vi "Burn-In Testing_v2.vi"() -> ()   [LabVIEW 2012]
uses:
  Controls/Command_Enum.ctl
  TestData/Command.ctl
  Controls/Exit.vi
  Classes/EpiWrapper.lvclass
  Controls/USB4000_Data.ctl
  Controls/Instr_Param.ctl
  Controls/PathTypes.ctl
  Controls/PathTraveler.ctl
  Controls/AppPaths.ctl
  Controls/PadArea.ctl
  Controls/Pad.ctl
  Controls/SelectedPads.ctl
  Controls/PadLookupItem.ctl
  Controls/PadLookup.ctl
  Controls/Measurement.ctl
  Controls/TestData.ctl
  Controls/MeasureControl.ctl
  Controls/MapEventType.ctl
  PadLookupVar.vi
  Controls/PadAreaItemStrings.ctl
  PadAreaStringsVar.vi
  Controls/UserInput.ctl
  Controls/MapPOS.ctl
  Controls/WaferTable.ctl
  Controls/Config.ctl
  Instruments/TypeDefs/SMUParam.ctl
  Controls/WaferSize.ctl
  Controls/CurrentPad.ctl
  Controls/MeasurementType.ctl
panel:
  in  "CurrentPad":T1
  in  "MeasureControl":T3 {"TestData"."50mA Data"."Reverse" format="%#_3g"; "TestData"."50mA Data"."Current,mA" format="%_6g"; "TestData"."50mA Data"."Knee Current" format="%#_3g"; "TestData"."50mA Data"."WL" format="%_6g"; "TestData"."50mA Data"."Voltage" format="%_6g"; "TestData"."50mA Data"."Power" format="%_5g"; "TestData"."20mA Data"."Reverse" format="%#_3g"; "TestData"."20mA Data"."Current,mA" format="%_6g"; "TestData"."20mA Data"."Knee Current" format="%#_3g"; "TestData"."20mA Data"."WL" format="%_6g"; "TestData"."20mA Data"."Voltage" format="%_6g"; "TestData"."20mA Data"."Power" format="%_5g"}
  in  "Tab Control":enum32{"Data 20mA", "Data 50mA"}(tab)
  in  "Wafer Data,20mA":T6
  in  "Wafer Data,50mA":T6
  in  "PadLookup":T7
  out "SelectedPads":T9
  out "2D Picture":picture
  out "SpectrumSat":bool
  in  "AppPaths":T11={"DataDir"={"Enum"=enum."DataDir", "FileName"="", "Exists?"=FALSE, "Path"=path ""}, "OmniDriver"={"Enum"=enum."OmniDriver", "FileName"="OmniDriver32.dll", "Exists?"=FALSE, "Path"=path ""}, "OmniDriverCommon"={"Enum"=enum."OmniDriver_Common", "FileName"="common32.dll", "Exists?"=FALSE, "Path"=path ""}, "Configuration"={"Enum"=enum."Configuration", "FileName"="TestConfiguration.cfg", "Exists?"=FALSE, "Path"=path ""}, "WaferImage"={"Enum"=enum."WaferImage", "FileName"="EPI_Wafer_Labels.jpg", "Exists?"=FALSE, "Path"=path ""}}
  in  "Configuration":T14={"IntTime"=100, "Samples"=3, "PowerMin"=300.0, "KneeMin"=-20.0, "KneeMax"=20.0, "Background Wl"=275.0, "Settle Delay,ms"=275, "StationId"=0.0} {"Background Wl" min=220.0 max=320.0; "IntTime" min=1 max=100000; "Samples" min=1 max=10; "PowerMin" min=0.0 max=10000.0; "KneeMin" min=-40.0 max=0.0; "KneeMax" min=0.0 max=40.0}
  out "Output For Excel":string
  in  "Integration Time(ms)\nMin=10ms":i32=10 min=10 max=100000
  out "Status":bool
  in  "MapPOS":T15
  in  "INSTR_PARAM":T16={"Keithley_Param"={"Start Current,mA"=0.0, "Stop Current,mA"=0.0, "Voltage Compliance,V"=0.0, "GPIB"="", "VISA resource name"="GPIB0::24::INSTR"}, "USB4000_Param"={"Integration Time"=0, "Wl min,nm"=0.0, "Wl max,nm"=0.0, "USB4000"={"Wrapper Out"=0, "Number of Spectrometers"=0, "Wavelength"=[], "EL Spectrum"=[], "Int Time (usec)"=0, FALSE, "Background"=[]}}, "Ophir_Param"={"VISA resource name"="", "Calibration Wl"=0.0}}
  in  "Stop":bool
  in  "Input":T19={"Wafer ID"="", "Test Type"=enum."Initial", "New"=FALSE, "Save"=FALSE, "Load"=FALSE, "Cancel"=FALSE, "Wafer Size"="2"}
  # "Quick Test"
  # "Measure Control"
  # "Measurement Settings"
  # "Test Criteria"
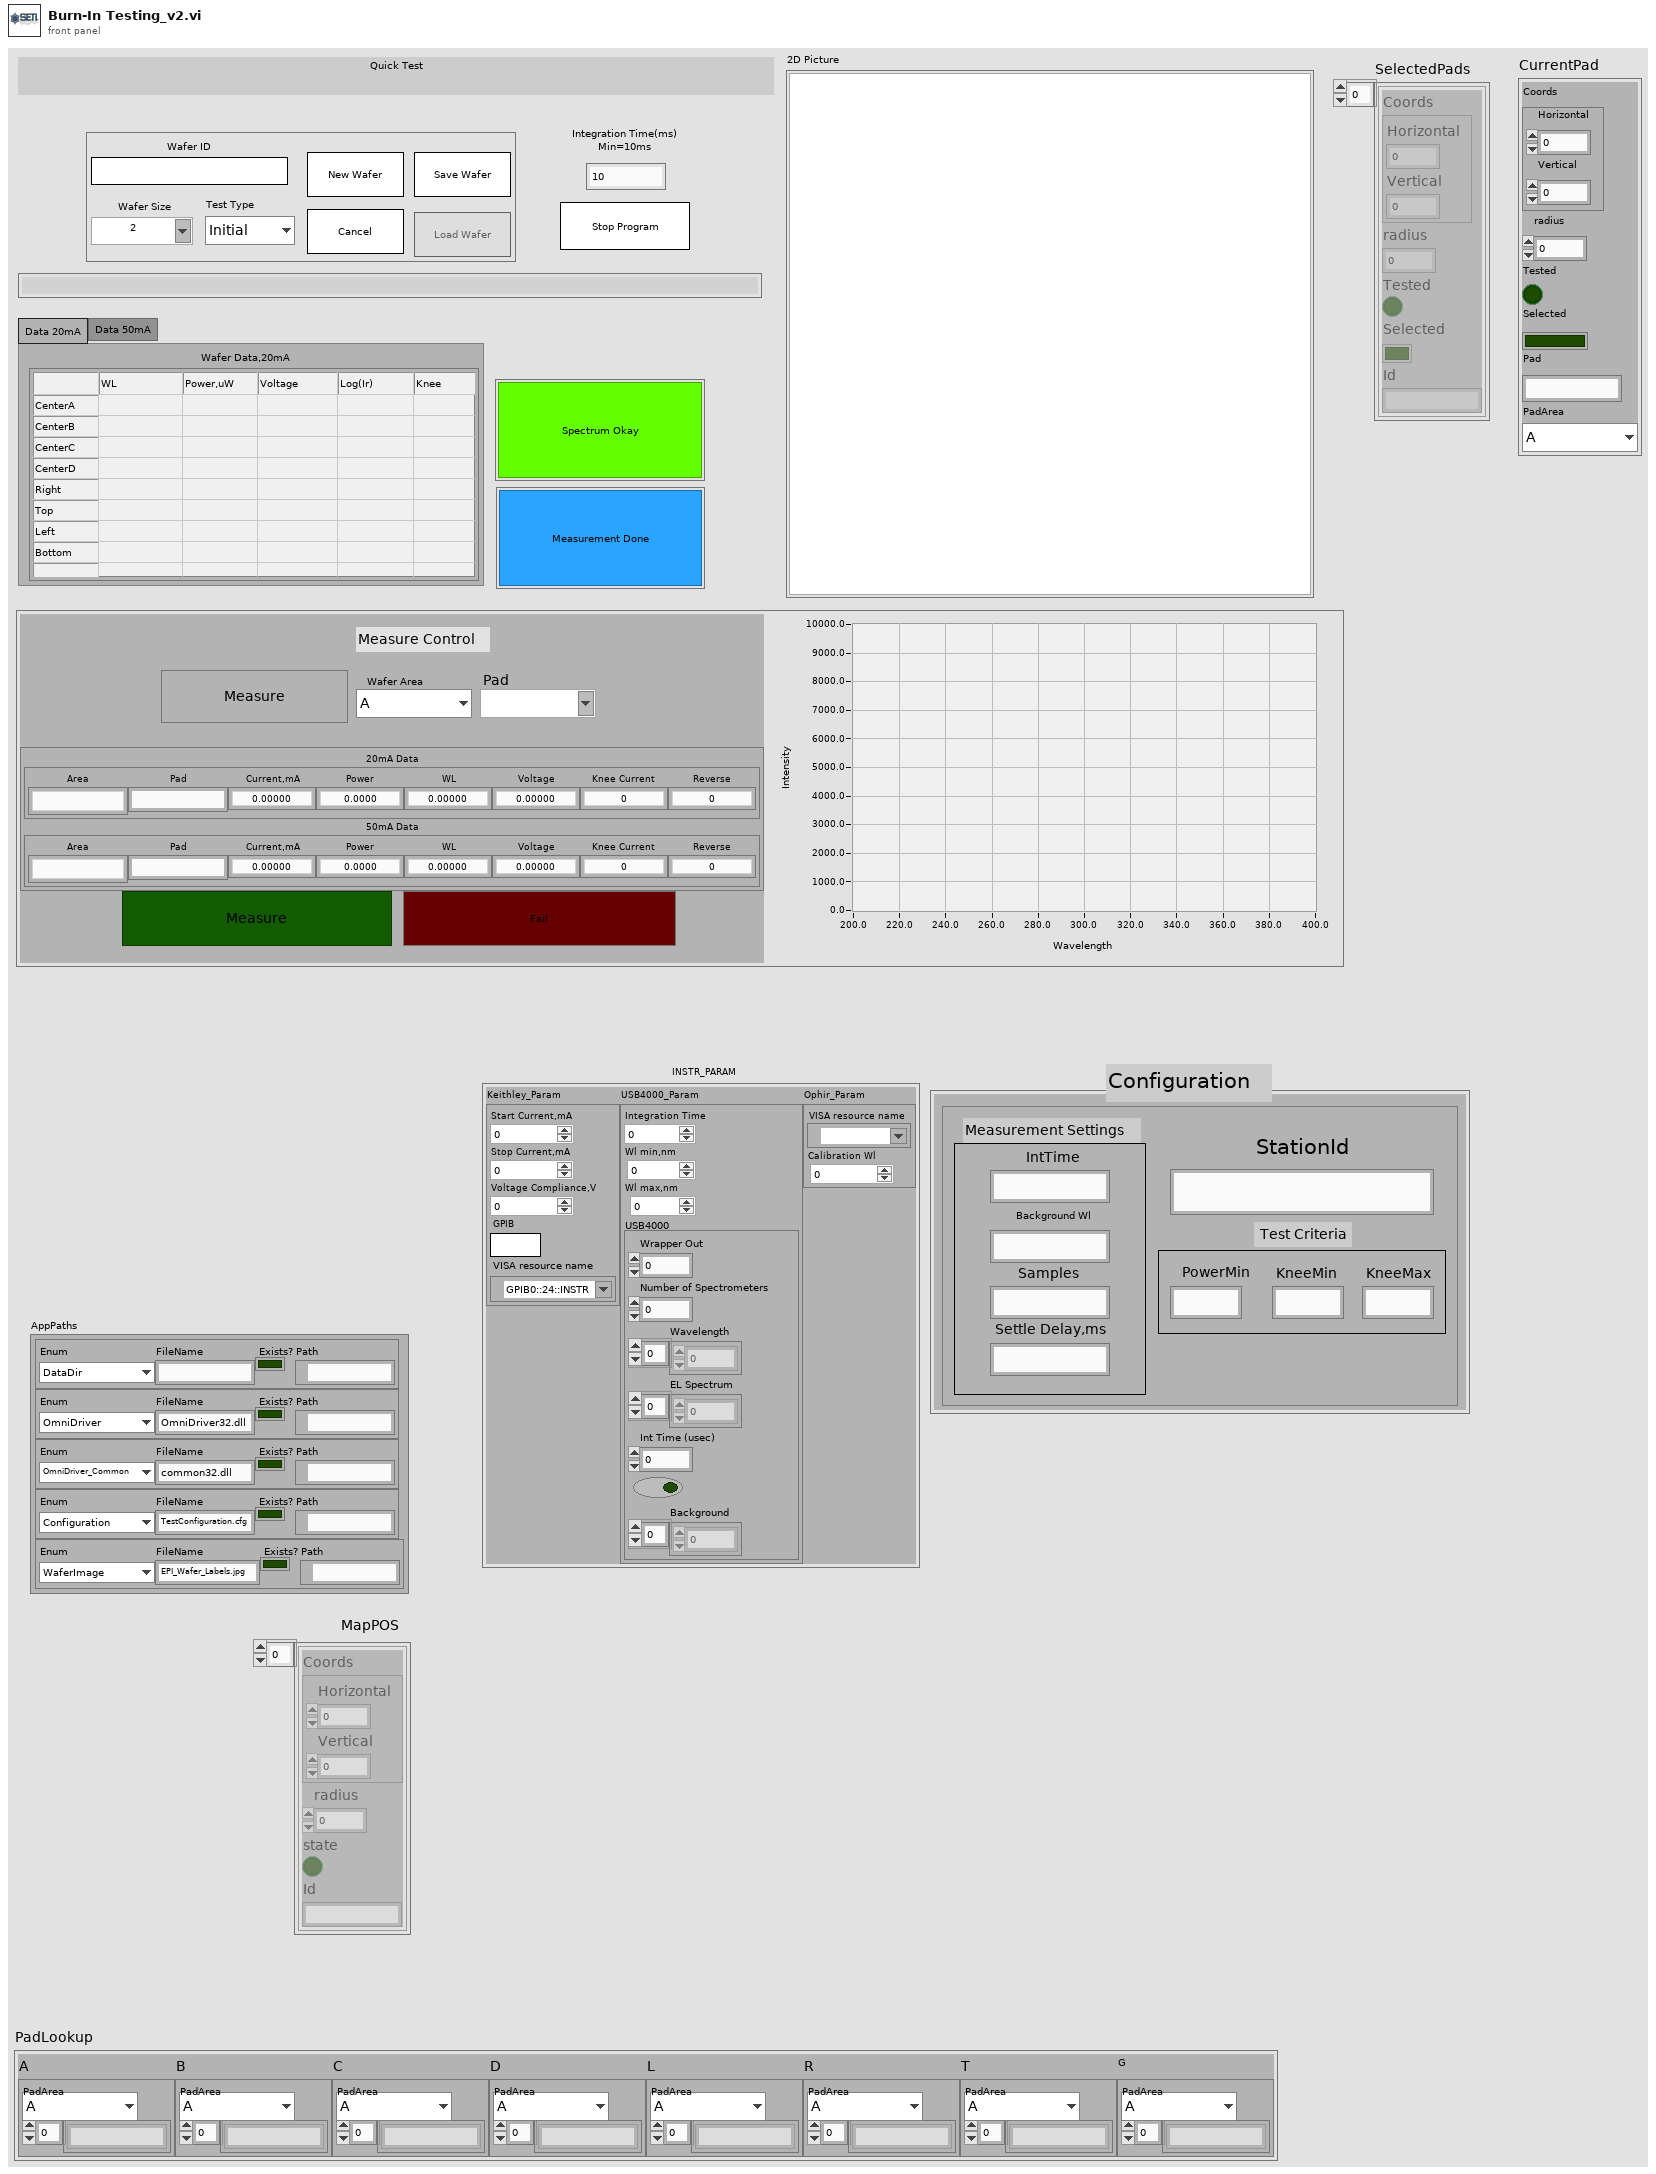
[diagram p1: front panel]
types:
  T1 = typedef "CurrentPad.ctl" = cluster{"Coords":cluster{"Horizontal":sgl, "Vertical":sgl}, "radius":i32, "Tested":bool, "Selected":bool, "Pad":string, "PadArea":T2}
  T2 = typedef "PadArea.ctl" = enum16{"A", "B", "C", "D", "L", "R", "T", "G"}
  T3 = typedef "MeasureControl.ctl" = cluster{"Graph":cluster{"Y":dbl[], "Y":dbl[]}[], "Pass":bool, "Fail":bool, "Measure":bool, "Wafer Area":T2, "TestData":T4, "Pad":string}
  T4 = typedef "TestData.ctl" = cluster{"20mA Data":T5, "50mA Data ":T5}
  T5 = typedef "Measurement.ctl" = cluster{"Area":string, "Pad":string, "Current,mA":dbl, "Power":dbl, "WL":dbl, "Voltage":dbl, "Knee Current":dbl, "Reverse":dbl}
  T6 = typedef "WaferTable.ctl" = string[][]
  T7 = typedef "PadLookup.ctl" = cluster{"A":T8, "B":T8, "C":T8, "D":T8, "L":T8, "R":T8, "T":T8, "G":T8}
  T8 = typedef "PadLookupItem.ctl" = cluster{"PadArea":T2, string[]}
  T9 = typedef "SelectedPads.ctl" = T10[]
  T10 = typedef "Pad.ctl" = cluster{"Coords":cluster{"Horizontal":sgl, "Vertical":sgl}, "radius":i32, "Tested":bool, "Selected":bool, "Id":string}
  T11 = typedef "AppPaths.ctl" = cluster{"DataDir":T12, "OmniDriver":T12, "OmniDriverCommon":T12, "Configuration":T12, "WaferImage":T12}
  T12 = typedef "PathTraveler.ctl" = cluster{"Enum":T13, "FileName":string, "Exists?":bool, "Path":path}
  T13 = typedef "PathTypes.ctl" = enum16{"DataDir", "OmniDriver", "OmniDriver_Common", "Configuration", "WaferImage"}
  T14 = typedef "Config.ctl" = cluster{"IntTime":i32, "Samples":i32, "PowerMin":dbl, "KneeMin":dbl, "KneeMax":dbl, "Background Wl":dbl, "Settle Delay,ms":u32, "StationId":sgl}
  T15 = typedef "MapPOS.ctl" = cluster{"Coords":cluster{"Horizontal":sgl, "Vertical":sgl}, "radius":i32, "state":bool, "Id":string}[]
  T16 = typedef "Instr_Param.ctl" = cluster{"Keithley_Param":T17, "USB4000_Param":cluster{"Integration Time":i32, "Wl min,nm":dbl, "Wl max,nm":dbl, "USB4000":T18}, "Ophir_Param":cluster{"VISA resource name":refnum<visa-resource-name>, "Calibration Wl":dbl}}
  T17 = typedef "SMUParam.ctl" = cluster{"Start Current,mA":dbl, "Stop Current,mA":dbl, "Voltage Compliance,V":dbl, "GPIB":string, "VISA resource name":refnum<visa-resource-name>}
  T18 = typedef "USB4000_Data.ctl" = cluster{"Wrapper Out":u32, "Number of Spectrometers":i32, "Wavelength":dbl[], "EL Spectrum":dbl[], "Int Time (usec)":i32, bool, "Background":dbl[]}
  T19 = typedef "UserInput.ctl" = cluster{"Wafer ID":string, "Test Type":T20, "New":bool, "Save":bool, "Load":bool, "Cancel":bool, "Wafer Size":T21}
  T20 = typedef "MeasurementType.ctl" = enum16{"Initial", "Final"}
  T21 = typedef "WaferSize.ctl" = string
  T22 = cluster{"Coords":cluster{"Horizontal":sgl, "Vertical":sgl}, "radius":i32, "state":bool, "Id":string}[]
  T23 = typedef "PadAreaItemStrings.ctl" = string[]
  T24 = cluster{"Coords":cluster{"Horizontal":sgl, "Vertical":sgl}, "radius":i32, "state":bool, "Id":string}
  T25 = typedef "Command.ctl" = cluster{"Command":T26, "Data":variant, "type":variant}
  T26 = typedef "Command_Enum.ctl" = enum16{"SPECTRUMCAPTURE", "INSITUMEASURE", "RESETCONFIG", "OPENCONFIG", "RESET", "INIT", "LOAD", "MEASURE", "NEW", "SAVE", "UPDATE_INT", "SWAP_MODE", "UPDATE_ACQ", "MARK_MAP_SELECT", "MARK_MAP", "EXIT", "CANCEL"}
  T27 = enum8{"Enabled", "Disabled", "Disabled and Grayed Out"}
  T28 = typedef "MapEventType.ctl" = enum16{"MouseClick", "DropDown"}
  T29 = typedef "LVMouseTypeDef.ctl" = cluster{"Mouse Position":cluster{"X":i32, "Y":i32}, "Mouse Modifiers":cluster{"Button Down":bool, "Shift Mod":bool, "Menu Mod":bool, "Option Mod":bool}}
  T30 = typedef "StartLotTraveler.ctl" = cluster{"Wafer ID":string, "Measurement Type":T20, "Exists?":bool, "Tested?":bool, "SameId?":bool}
  T31 = typedef "LVPoint32TypeDef.ctl" = cluster{"Horizontal":i32, "Vertical":i32}
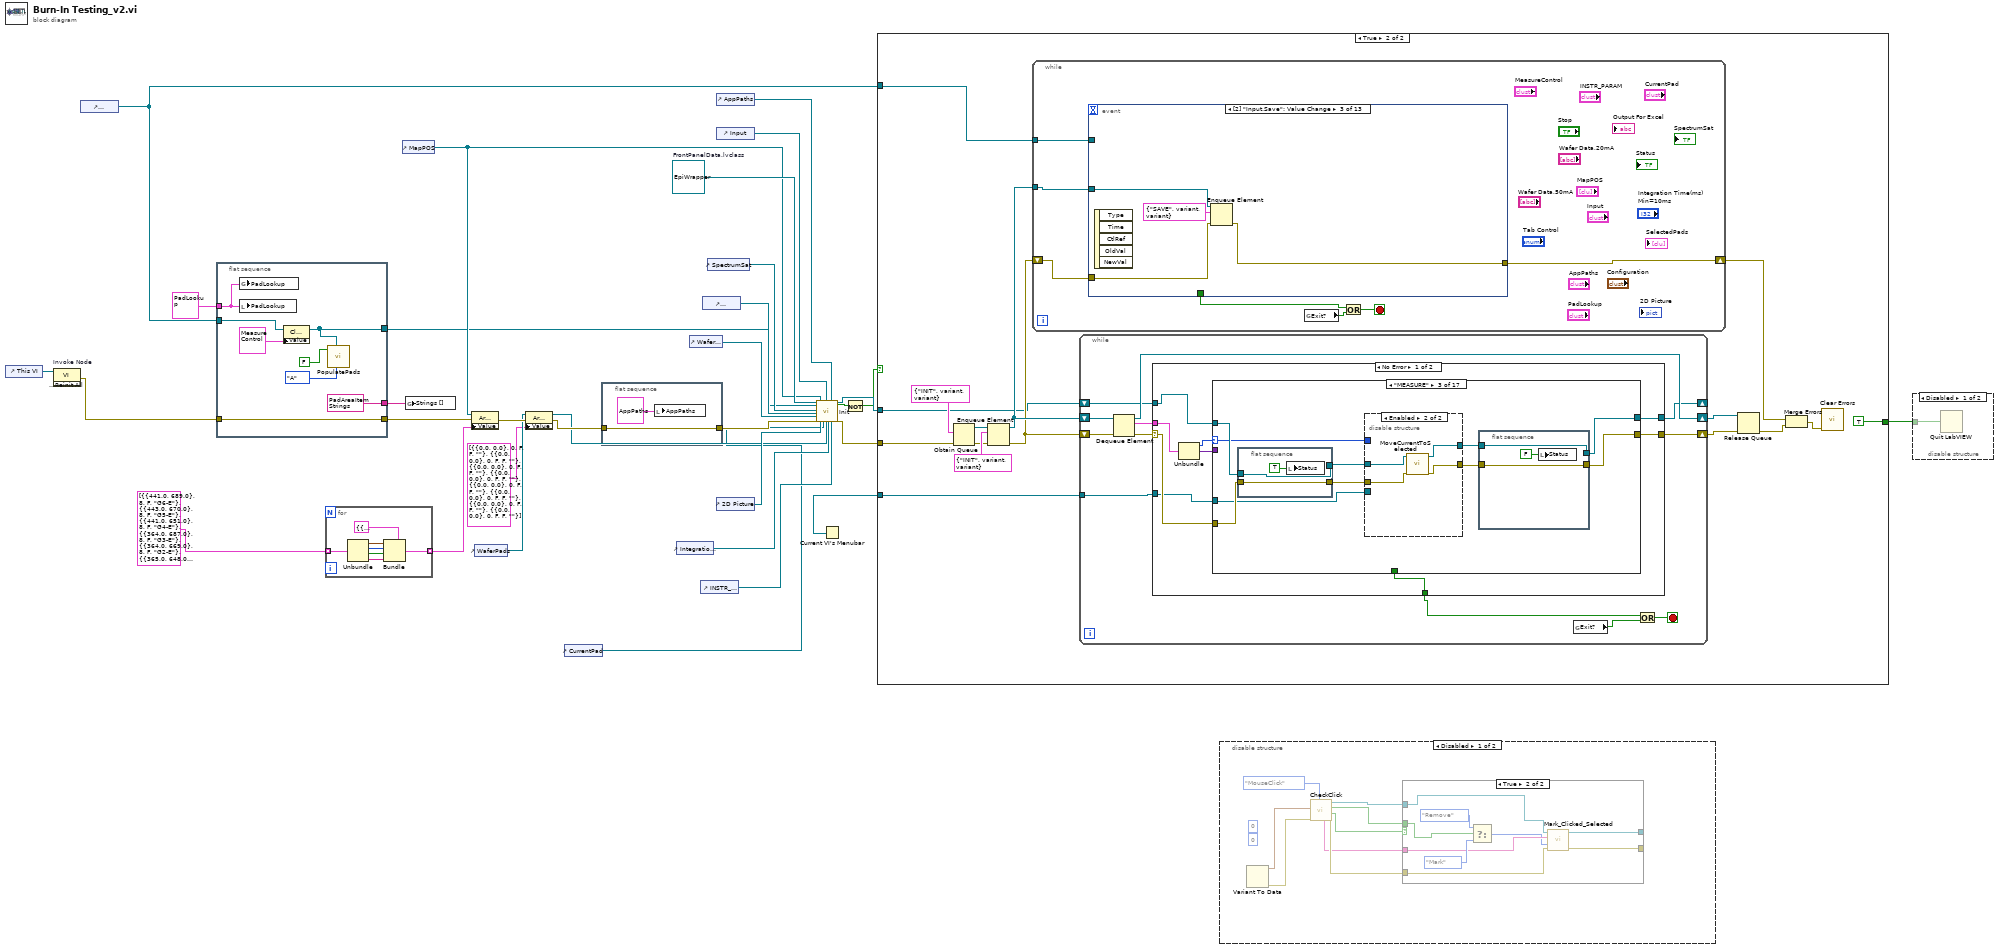
[diagram p0: block diagram]
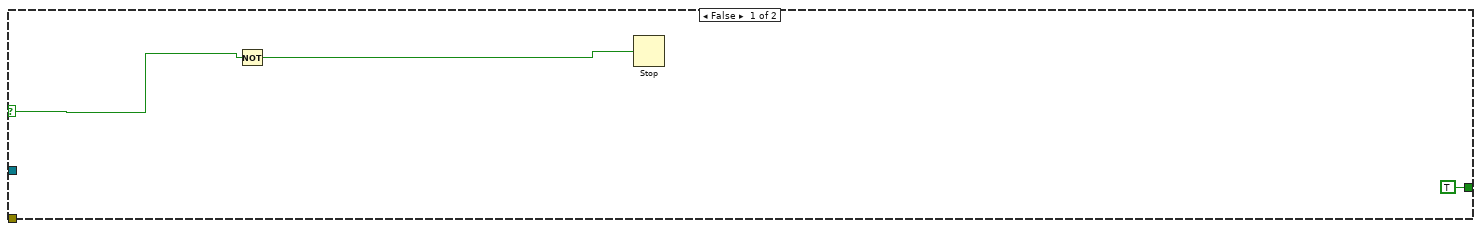
[diagram p5: hidden frame]
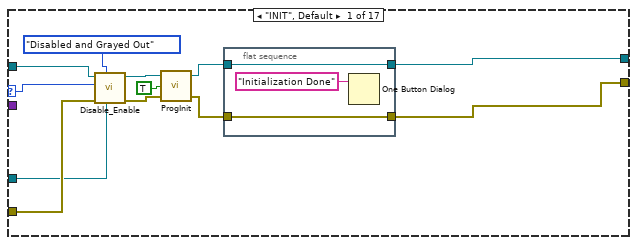
[diagram p6: hidden frame]
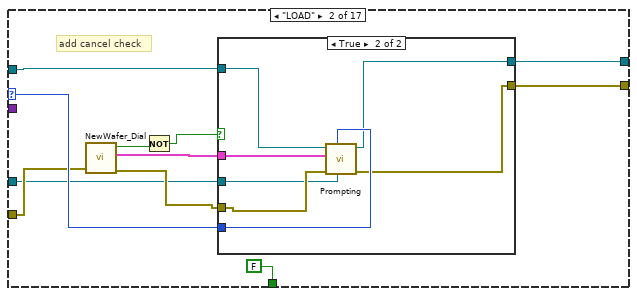
[diagram p7: hidden frame]
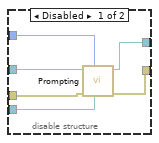
[diagram p9: hidden frame]
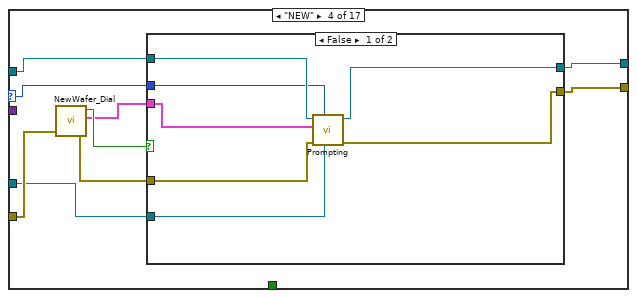
[diagram p10: hidden frame]
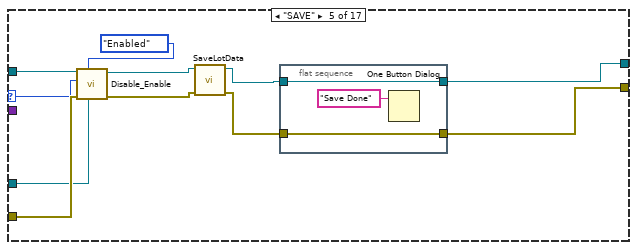
[diagram p12: hidden frame]
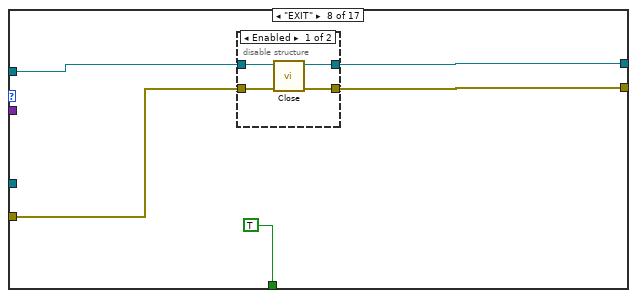
[diagram p15: hidden frame]
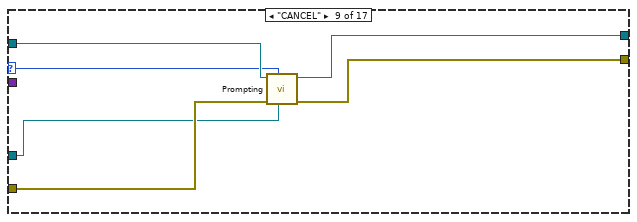
[diagram p17: hidden frame]
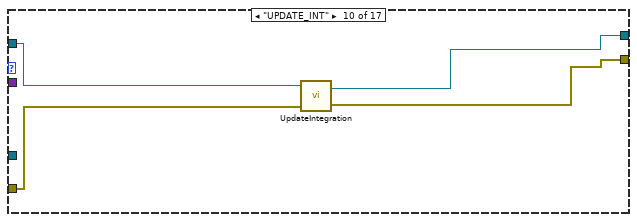
[diagram p18: hidden frame]
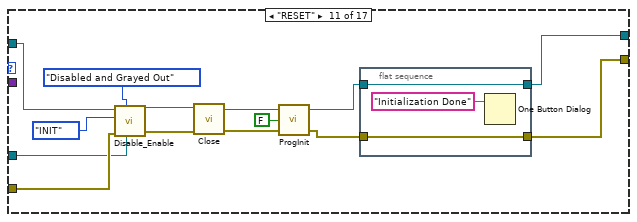
[diagram p19: hidden frame]
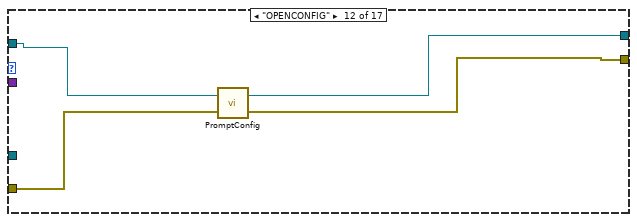
[diagram p20: hidden frame]
diagram:
  w32 = refnum<class "EpiWrapper.lvclass"> refnum  # FrontPanelData.lvclass
  n1 = control-ref of="This VI"() -> (w29:refnum<vi>)
  n2 = invoke on="Invoke Node" class="VI" method="Default Vals.Reinit All"(reference=w29) -> (error out=w3:errorcluster)  [unwired: 2 in, 2 out]
  n3 = control-ref of="MeasureControl"() -> (w7:refnum<vi>)
  n4 = flat-sequence {
    tunnel: w7 -> [w40]
    tunnel: [w34] -> w6
    tunnel: T7 {"A"={"PadArea"=enum."A", ["A"]}, "B"={"PadArea"=enum."B", ["B"]}, "C"={"PadArea"=enum."C", ["C"]}, "D"={"PadArea"=enum."D", ["C"]}, "L"={"PadArea"=enum."L", ["L1-E", "L2-E", "L3-E", "L4-E", "L5-E", "L6-E"]}, "R"={"PadArea"=enum."R", ["R1-E", "R2-E", "R3-E", "R4-E", "R5-E", "R6-E"]}, "T"={"PadArea"=enum."T", ["T1-E", "T2-E", "T3-E", "T4-E", "T5-E", "T6-E"]}, "G"={"PadArea"=enum."G", ["G1-E", "G2-E", "G3-E", "G4-E", "G5-E", "G6-E"]}} ("PadLookup") -> [w35]
    tunnel: [w36] -> w4
    tunnel: w3 -> [w36]
    tunnel: [T23 ["A", "B", "C", "D", "L", "R", "T", "G"] ("Strings []")] -> w1
    frame #0 {
      n5 = global write "PadLookupVar.vi" "PadLookup"(w35) -> ()
      n6 = local write "PadLookup"(w35) -> ()
      n7 = property class="Clust (strict)"(reference=w40, "Value"=T3 {"Graph"=[], "Pass"=FALSE, "Fail"=FALSE, "Measure"=FALSE, "Wafer Area"=enum."A", "TestData"={"20mA Data"={"Area"="", "Pad"="", "Current,mA"=0.0, "Power"=0.0, "WL"=0.0, "Voltage"=0.0, "Knee Current"=0.0, "Reverse"=0.0}, "50mA Data "={"Area"="", "Pad"="", "Current,mA"=0.0, "Power"=0.0, "WL"=0.0, "Voltage"=0.0, "Knee Current"=0.0, "Reverse"=0.0}}, "Pad"=""}) -> (reference out=w34:refnum<vi>)  [unwired: 1 in, 1 out]
      n8 = call "PopulatePads.vi"("Set Pad?"=FALSE, "MeasureControl"=w34, "PadArea"=PadArea."A") -> ()  [unwired: 3 in]
    }
  }
  n9 = for {
    tunnel: T22 [{"Coords"={"Horizontal"=441.0, "Vertical"=689.0}, "radius"=8, "state"=FALSE, "Id"="G6-E"}, {"Coords"={"Horizontal"=443.0, "Vertical"=670.0}, "radius"=8, "state"=FALSE, "Id"="G5-E"}, {"Coords"={"Horizontal"=441.0, "Vertical"=651.0}, "radius"=8, "state"=FALSE, "Id"="G4-E"}, {"Coords"={"Horizontal"=364.0, "Vertical"=687.0}, "radius"=8, "state"=FALSE, "Id"="G3-E"}, {"Coords"={"Horizontal"=364.0, "Vertical"=669.0}, "radius"=8, "state"=FALSE, "Id"="G2-E"}, {"Coords"={"Horizontal"=365.0, "Vertical"=648.0}, "radius"=9, "state"=FALSE, "Id"="G1-E"}, {"Coords"={"Horizontal"=672.0, "Vertical"=446.0}, "radius"=8, "state"=FALSE, "Id"="R6-E"}, {"Coords"={"Horizontal"=652.0, "Vertical"=445.0}, "radius"=8, "state"=FALSE, "Id"="R5-E"}, {"Coords"={"Horizontal"=633.0, "Vertical"=445.0}, "radius"=9, "state"=FALSE, "Id"="R4-E"}, {"Coords"={"Horizontal"=669.0, "Vertical"=374.0}, "radius"=8, "state"=FALSE, "Id"="R3-E"}, {"Coords"={"Horizontal"=651.0, "Vertical"=373.0}, "radius"=8, "state"=FALSE, "Id"="R2-E"}, {"Coords"={"Horizontal"=633.0, "Vertical"=374.0}, "radius"=9, "state"=FALSE, "Id"="R1-E"}, {"Coords"={"Horizontal"=446.0, "Vertical"=125.0}, "radius"=8, "state"=FALSE, "Id"="T6-E"}, {"Coords"={"Horizontal"=447.0, "Vertical"=144.0}, "radius"=8, "state"=FALSE, "Id"="T5-E"}, {"Coords"={"Horizontal"=445.0, "Vertical"=163.0}, "radius"=8, "state"=FALSE, "Id"="T4-E"}, {"Coords"={"Horizontal"=365.0, "Vertical"=127.0}, "radius"=8, "state"=FALSE, "Id"="T3-E"}, {"Coords"={"Horizontal"=364.0, "Vertical"=145.0}, "radius"=8, "state"=FALSE, "Id"="T2-E"}, {"Coords"={"Horizontal"=364.0, "Vertical"=164.0}, "radius"=8, "state"=FALSE, "Id"="T1-E"}, {"Coords"={"Horizontal"=180.0, "Vertical"=442.0}, "radius"=8, "state"=FALSE, "Id"="L6-E"}, {"Coords"={"Horizontal"=161.0, "Vertical"=441.0}, "radius"=8, "state"=FALSE, "Id"="L5-E"}, {"Coords"={"Horizontal"=141.0, "Vertical"=442.0}, "radius"=9, "state"=FALSE, "Id"="L4-E"}, {"Coords"={"Horizontal"=179.0, "Vertical"=365.0}, "radius"=8, "state"=FALSE, "Id"="L3-E"}, {"Coords"={"Horizontal"=162.0, "Vertical"=365.0}, "radius"=9, "state"=FALSE, "Id"="L2-E"}, {"Coords"={"Horizontal"=142.0, "Vertical"=364.0}, "radius"=9, "state"=FALSE, "Id"="L1-E"}, {"Coords"={"Horizontal"=444.0, "Vertical"=363.0}, "radius"=8, "state"=FALSE, "Id"="C"}, {"Coords"={"Horizontal"=444.0, "Vertical"=441.0}, "radius"=8, "state"=FALSE, "Id"="B"}, {"Coords"={"Horizontal"=368.0, "Vertical"=442.0}, "radius"=9, "state"=FALSE, "Id"="A"}, {"Coords"={"Horizontal"=368.0, "Vertical"=364.0}, "radius"=9, "state"=FALSE, "Id"="D"}] ("Adjusted") -> [w46] mode=indexing
    tunnel: [w41] -> w15 mode=indexing
    n10 = Unbundle(w46) -> ("Coords"=w45:cluster{"Horizontal":sgl, "Vertical":sgl}, "radius"=w44:i32, "state"=w42:bool, "Id"=w43:string)
    n11 = Bundle(cluster=T24 {"Coords"={"Horizontal"=0.0, "Vertical"=0.0}, "radius"=0, "state"=FALSE, "Id"=""} ("output cluster"), "Coords"=w45, "radius"=w44, "state"=w42, "Id"=w43) -> (w41:T24)
  }
  n12 = control-ref of="MapPOS"() -> (w12:refnum<vi>)
  n13 = global write "PadAreaStringsVar.vi" "Strings []"(w1) -> ()
  n14 = property class="Arr (strict)"(reference=w12, error in=w4, "Value"=w15) -> (error out=w14:errorcluster)  [unwired: 1 out]
  n15 = control-ref of="WaferPads"() -> (w13:refnum<vi>)
  n16 = property class="Arr (strict)"(reference=w13, error in=w14, "Value"=T9 [{"Coords"={"Horizontal"=0.0, "Vertical"=0.0}, "radius"=0, "Tested"=FALSE, "Selected"=FALSE, "Id"=""}, {"Coords"={"Horizontal"=0.0, "Vertical"=0.0}, "radius"=0, "Tested"=FALSE, "Selected"=FALSE, "Id"=""}, {"Coords"={"Horizontal"=0.0, "Vertical"=0.0}, "radius"=0, "Tested"=FALSE, "Selected"=FALSE, "Id"=""}, {"Coords"={"Horizontal"=0.0, "Vertical"=0.0}, "radius"=0, "Tested"=FALSE, "Selected"=FALSE, "Id"=""}, {"Coords"={"Horizontal"=0.0, "Vertical"=0.0}, "radius"=0, "Tested"=FALSE, "Selected"=FALSE, "Id"=""}, {"Coords"={"Horizontal"=0.0, "Vertical"=0.0}, "radius"=0, "Tested"=FALSE, "Selected"=FALSE, "Id"=""}, {"Coords"={"Horizontal"=0.0, "Vertical"=0.0}, "radius"=0, "Tested"=FALSE, "Selected"=FALSE, "Id"=""}, {"Coords"={"Horizontal"=0.0, "Vertical"=0.0}, "radius"=0, "Tested"=FALSE, "Selected"=FALSE, "Id"=""}] ("WaferPads 2")) -> (reference out=w8:refnum<vi>, error out=w11:errorcluster)
  n17 = control-ref of="CurrentPad"() -> (w2:refnum<vi>)
  n18 = flat-sequence {
    tunnel: w11 -> [w49]
    tunnel: [w49] -> w25
    frame #0 {
      n19 = local write "AppPaths"(T11 {"DataDir"={"Enum"=enum."DataDir", "FileName"="", "Exists?"=FALSE, "Path"=path ""}, "OmniDriver"={"Enum"=enum."OmniDriver", "FileName"="OmniDriver32.dll", "Exists?"=FALSE, "Path"=path ""}, "OmniDriverCommon"={"Enum"=enum."OmniDriver_Common", "FileName"="common32.dll", "Exists?"=FALSE, "Path"=path ""}, "Configuration"={"Enum"=enum."Configuration", "FileName"="TestConfiguration.cfg", "Exists?"=FALSE, "Path"=path ""}, "WaferImage"={"Enum"=enum."WaferImage", "FileName"="EPI_Wafer_Labels.jpg", "Exists?"=FALSE, "Path"=path ""}} ("AppPaths")) -> ()
    }
  }
  n20 = control-ref of="Integration Time(ms)\nMin=10ms"() -> (w26:refnum<vi>)
  n21 = control-ref of="Wafer Data,20mA"() -> (w20:refnum<vi>)
  n22 = control-ref of="INSTR_PARAM"() -> (w21:refnum<vi>)
  n23 = control-ref of="Configuration"() -> (w19:refnum<vi>)
  n24 = control-ref of="SpectrumSat"() -> (w18:refnum<vi>)
  n25 = control-ref of="AppPaths"() -> (w24:refnum<vi>)
  n26 = control-ref of="Input"() -> (w17:refnum<vi>)
  n27 = control-ref of="2D Picture"() -> (w16:refnum<vi>)
  n28 = call-dynamic "Init.vi"("FrontPanelData in"=w32, "MeasureControl"=w6, "SpectrumSat"=w18, "Configuration"=w19, "WaferTable_Ref"=w20, "error in (no error)"=w25, "MapPositions"=w12, "WaferMao"=w16, "CurrentPad"=w2, "Input"=w17, "WaferPads"=w8, "IntTime_Ref"=w26, "AppPaths"=w24, "INSTR_PARAM"=w21) -> ("FrontPanelData out"=w31:refnum<class "EpiWrapper.lvclass">, "Shutdown?"=w28:bool, "error out"=w30:errorcluster)  [unwired: 11 in]
  n29 = Current VI's Menubar() -> (w22:refnum<k9>)
  n30 = Not(x=w28) -> (.not. x?=w27:bool)
  n31 = case shown="True" w27 {
    selector: w27 -> [w51 _]
    tunnel: w31 -> [_ w63]
    tunnel: w30 -> [_ w62]
    tunnel: [TRUE ("quit? (T)") TRUE ("quit? (T)")] -> w23
    tunnel: w22 -> [_ w54]
    tunnel: w7 -> [_ w53]
    frame False {
      n32 = Not(x=w51) -> (.not. x?=w50:bool)
      n33 = Stop(stop? (T)=w50) -> ()
    }
    frame True {
      n34 = Obtain Queue(element data type=T25 {"Command"=enum."INIT", "Data"=variant, "type"=variant} ("Cluster"), error in (no error)=w62) -> (queue out=w66:refnum<queue>, error out=w61:errorcluster)  [unwired: 3 in, 1 out]
      n35 = Enqueue Element(queue=w66, element=T25 {"Command"=enum."INIT", "Data"=variant, "type"=variant}, error in (no error)=w61) -> (queue out=w68:refnum<queue>, error out=w64:errorcluster)  [unwired: 1 in, 1 out]
      n36 = while {
        tunnel: w68 -> [w272]
        shift-right: [w267] -> w56
        shift-left: w64 -> [w268]
        tunnel: w53 -> [w266]
        stop <- w270 stop-if-true
        n37 = event shown="[2] \"Input.Save\": Value Change" {
          selector: _ -> [_ _ _ _ _ _ _ _ _ _ _ _ _]
          dyn-events: _ -> [_ _ _ _ _ _ _ _ _ _ _ _ _]
          timeout: _ -> [_ _ _ _ _ _ _ _ _ _ _ _ _]
          tunnel: w272 -> [_ w277 w281 w286 w289 w293 w297 w302 w343 w346 _ w356 w360]
          tunnel: [_ TRUE ("x") _ _ _ _ _ w299 _ _ _ TRUE ("x") _] -> w269
          tunnel: w268 -> [w273 w275 w280 w285 w288 w292 w296 w301 w342 _ w349 w355 w359]
          tunnel: [w273 w274 w279 w283 w287 w294 w295 w300 w341 w345 w349 w353 w358] -> w267
          tunnel: w266 -> [_ _ _ _ _ _ _ _ _ _ w350 _ _]
          event Timeout {
            n38 = event-data() -> ()  [unwired: 1 in, 2 out]
          }
          event "Stop": Value Change {
            n39 = event-data() -> ()  [unwired: 1 in, 5 out]
            n40 = Enqueue Element(queue=w277, element=T25 {"Command"=enum."EXIT", "Data"=variant, "type"=variant}, error in (no error)=w275) -> (error out=w274:errorcluster)  [unwired: 1 in, 2 out]
          }
          event Value Change {
            n41 = event-data() -> ()  [unwired: 1 in, 5 out]
            n42 = Enqueue Element(queue=w281, element=T25 {"Command"=enum."SAVE", "Data"=variant, "type"=variant}, error in (no error)=w280) -> (error out=w279:errorcluster)  [unwired: 1 in, 2 out]
          }
          event Value Change {
            n43 = event-data() -> ()  [unwired: 1 in, 5 out]
            n44 = Enqueue Element(queue=w286, element=T25 {"Command"=enum."MEASURE", "Data"=variant, "type"=variant}, error in (no error)=w285) -> (error out=w283:errorcluster)  [unwired: 1 in, 2 out]
          }
          event Value Change {
            n45 = event-data() -> ()  [unwired: 1 in, 5 out]
            n46 = Enqueue Element(queue=w289, element=T25 {"Command"=enum."CANCEL", "Data"=variant, "type"=variant}, error in (no error)=w288) -> (error out=w287:errorcluster)  [unwired: 1 in, 2 out]
          }
          event Value Change {
            n47 = event-data() -> ()  [unwired: 1 in, 5 out]
            n48 = Enqueue Element(queue=w293, element=T25 {"Command"=enum."NEW", "Data"=variant, "type"=variant}, error in (no error)=w292) -> (error out=w294:errorcluster)  [unwired: 1 in, 2 out]
          }
          event Value Change {
            n49 = event-data() -> ()  [unwired: 1 in, 5 out]
            n50 = Enqueue Element(queue=w297, element=T25 {"Command"=enum."LOAD", "Data"=variant, "type"=variant}, error in (no error)=w296) -> (error out=w295:errorcluster)  [unwired: 1 in, 2 out]
          }
          event Menu Selection (User) {
            n51 = event-data() -> ("ItemTag"=w303:string)  [unwired: 1 in]
            n52 = case shown="\"INSITUMEASURE\"" w303 {
              tunnel: w302 -> [_ w309 w312 w319 w324 w330 w334]
              tunnel: w301 -> [w305 w308 w313 w318 w323 w328 w332]
              tunnel: [w305 w307 w314 w317 w322 w327 w333] -> w300
              tunnel: [FALSE ("x") FALSE ("x") TRUE ("x") FALSE ("x") FALSE ("x") FALSE ("x") FALSE ("x")] -> w299
              frame "False", Default {
              }
              frame "OPENCONFIG" {
                n53 = Enqueue Element(queue=w309, element=T25 {"Command"=enum."OPENCONFIG", "Data"=variant, "type"=variant}, error in (no error)=w308) -> (error out=w307:errorcluster)  [unwired: 1 in, 2 out]
              }
              frame "EXIT" {
                n54 = Enqueue Element(queue=w312, element=T25 {"Command"=enum."EXIT", "Data"=variant, "type"=variant}, error in (no error)=w313) -> (error out=w314:errorcluster)  [unwired: 1 in, 2 out]
              }
              frame "RESET" {
                n55 = Enqueue Element(queue=w319, element=T25 {"Command"=enum."RESET", "Data"=variant, "type"=variant}, error in (no error)=w318) -> (error out=w317:errorcluster)  [unwired: 1 in, 2 out]
              }
              frame "RESETCONFIG" {
                n56 = Enqueue Element(queue=w324, element=T25 {"Command"=enum."RESETCONFIG", "Data"=variant, "type"=variant}, error in (no error)=w323) -> (error out=w322:errorcluster)  [unwired: 1 in, 2 out]
              }
              frame "SPECTRUMCAPTURE" {
                n57 = Enqueue Element(queue=w330, element=T25 {"Command"=enum."SPECTRUMCAPTURE", "Data"=variant, "type"=variant}, error in (no error)=w328) -> (error out=w327:errorcluster)  [unwired: 1 in, 2 out]
              }
              frame "INSITUMEASURE" {
                n58 = Enqueue Element(queue=w334, element=T25 {"Command"=enum."INSITUMEASURE", "Data"=variant, "type"=variant}, error in (no error)=w332) -> (error out=w333:errorcluster)  [unwired: 1 in, 2 out]
              }
            }
          }
          event "2D Picture": Mouse Down {
            n59 = event-data() -> ("CtlRef"=w338:refnum<vi>)  [unwired: 1 in]
            n60 = property class="Pict"(reference=w338) -> ("Mouse"=w337:T29)  [unwired: 1 in, 2 out]
            n61 = Unbundle By Name(w337) -> ("Mouse Position"=w336:cluster{"X":i32, "Y":i32})
            n62 = Bundle By Name(cluster=T25 {"Command"=enum."MARK_MAP", "Data"=variant, "type"=variant} ("element"), "Data"=w336) -> (w339:T25)
            n63 = Enqueue Element(queue=w343, element=w339, error in (no error)=w342) -> (error out=w341:errorcluster)  [unwired: 1 in, 2 out]
          }
          event Value Change {
            n64 = event-data() -> ("NewVal"=w344:string)  [unwired: 1 in, 2 out]
            n65 = Bundle By Name(cluster=T25 {"Command"=enum."MARK_MAP_SELECT", "Data"=variant, "type"=variant} ("element"), "Data"=w344) -> (w347:T25)
            n66 = Enqueue Element(queue=w346, element=w347) -> (error out=w345:errorcluster)  [unwired: 2 in, 2 out]
          }
          event Value Change {
            n67 = event-data() -> ("NewVal"=w352:T2)  [unwired: 1 in, 2 out]
            n68 = call "PopulatePads.vi"("Set Pad?"=FALSE, "MeasureControl"=w350, "PadArea"=w352) -> ()  [unwired: 3 in]
          }
          event Panel Close {
            n69 = event-data() -> ()  [unwired: 1 in, 4 out]
            n70 = Enqueue Element(queue=w356, element=T25 {"Command"=enum."EXIT", "Data"=variant, "type"=variant}, error in (no error)=w355) -> (error out=w353:errorcluster)  [unwired: 1 in, 2 out]
          }
          event "Integration Time(ms)\nMin=10ms": Value Change {
            n71 = event-data() -> ()  [unwired: 1 in, 5 out]
            n72 = Enqueue Element(queue=w360, element=T25 {"Command"=enum."UPDATE_INT", "Data"=variant, "type"=variant}, error in (no error)=w359) -> (error out=w358:errorcluster)  [unwired: 1 in, 2 out]
          }
        }
        n73 = global read "Exit.vi" "Exit?"() -> (w271:bool)
        n74 = Or(x=w269, y=w271) -> (x .or. y?=w270:bool)
      }
      n75 = while {
        shift-right: [w76] -> w60
        shift-left: w68 -> [w80]
        shift-right: [w77] -> w59
        shift-left: w64 -> [w78]
        shift-right: [w70] -> _
        shift-left: w63 -> [w71]
        tunnel: w54 -> [w69]
        stop <- w73 stop-if-true
        n76 = Dequeue Element(queue=w80, error in (no error)=w78) -> (queue out=w76:refnum<queue>, element=w75:T25, error out=w79:errorcluster)  [unwired: 1 in, 1 out]
        n77 = case shown="No Error" w79 {
          selector: w79 -> [w85 w264]
          tunnel: [w86 w263] -> w77
          tunnel: w75 -> [w89 _]
          tunnel: [w87 _] -> w72
          tunnel: w71 -> [w84 w265]
          tunnel: [w83 w265] -> w70
          tunnel: w69 -> [w81 _]
          frame No Error {
            n78 = Unbundle(w89) -> ("Command"=w88:T26, "Data"=w82:variant)  [unwired: 1 out]
            n79 = case shown="\"MEASURE\"" w88 {
              selector: w88 -> [w94 w110 w128 w151 w170 _ _ _ w199 _ _ _ _ w234 w239 _ _]
              tunnel: [_ FALSE ("y") _ _ _ _ _ TRUE ("y") _ _ _ _ _ _ _ _ _] -> w87
              tunnel: [w92 w111 w125 w155 w172 w184 w186 w187 w201 w204 w211 w227 w230 w236 w242 w245 w254] -> w86
              tunnel: w85 -> [w98 w107 w133 w154 w178 w184 w186 w189 w202 w206 w219 w225 w231 w237 w241 w252 w262]
              tunnel: w84 -> [w99 w113 w134 w157 w179 w183 w185 w190 w203 w207 w220 w228 w232 w238 w244 w250 w259]
              tunnel: [w93 w112 w130 w156 w171 w183 w185 w188 w200 w205 w210 w226 w229 w235 w243 w246 w255] -> w83
              tunnel: w82 -> [_ _ _ _ _ _ _ _ _ _ _ _ _ _ _ w253 w261]
              tunnel: w81 -> [w91 w105 w126 w152 w169 _ _ _ w198 _ w209 _ _ w233 w240 _ _]
              frame "INIT", Default {
                n80 = call-dynamic "Disable_Enable.vi"("menu reference"=w91, "Disabled"=T27."Disabled and Grayed Out", "error in (no error)"=w98, "Command"=w94, "EpiWrapper in"=w99) -> ("error out"=w96:errorcluster, "EpiWrapper out"=w97:refnum<class "EpiWrapper.lvclass">)  [unwired: 5 in]
                n81 = call-dynamic "ProgInit.vi"("error in (no error)"=w96, "Intialize?"=TRUE, "EpiWrapper in"=w97) -> ("error out"=w101:errorcluster, "EpiWrapper out"=w100:refnum<class "EpiWrapper.lvclass">)  [unwired: 1 in]
                n82 = flat-sequence {
                  tunnel: [w103] -> w92
                  tunnel: w101 -> [w103]
                  tunnel: [w102] -> w93
                  tunnel: w100 -> [w102]
                  frame #0 {
                    n83 = One Button Dialog(message="Initialization Done") -> ()  [unwired: 1 in, 1 out]
                  }
                }
              }
              frame "LOAD" {
                # "add cancel check"
                n84 = call "NewWafer_Dial.vi"("error in (no error)"=w107) -> ("Cancelled?"=w109:bool, "StartLotTraveler"=w114:T30, "error out"=w106:errorcluster)  [unwired: 3 in]
                n85 = Not(x=w109) -> (.not. x?=w108:bool)
                n86 = case shown="True" w108 {
                  tunnel: w114 -> [_ w118]
                  tunnel: w106 -> [w116 w122]
                  tunnel: w113 -> [w117 w124]
                  tunnel: [w117 w121] -> w112
                  tunnel: [w116 w120] -> w111
                  tunnel: w110 -> [_ w123]
                  tunnel: w105 -> [_ w119]
                  frame False {
                  }
                  frame True {
                    n87 = call-dynamic "Prompting.vi"("menu reference"=w119, "Command"=w123, "error in (no error)"=w122, "StartLotTraveler"=w118, "EpiWrapper in"=w124) -> ("error out"=w120:errorcluster, "EpiWrapper out"=w121:refnum<class "EpiWrapper.lvclass">)  [unwired: 5 in]
                  }
                }
              }
              frame "MEASURE" {
                n88 = flat-sequence {
                  tunnel: [w149] -> w132
                  tunnel: w134 -> [w149]
                  tunnel: w133 -> [w148]
                  tunnel: [w148] -> w127
                  frame #0 {
                    n89 = local write "Status"(TRUE ("Status")) -> ()
                  }
                }
                n90 = disable-structure shown="Enabled" {
                  disable-tunnel: w132 -> [w140 w144]
                  disable-tunnel: [w139 w142] -> w131
                  disable-tunnel: [w138 w141] -> w129
                  disable-tunnel: w128 -> [w137 _]
                  disable-tunnel: w127 -> [w136 w143]
                  disable-tunnel: w126 -> [w135 _]
                  frame Disabled {
                    n91 = call-dynamic "Prompting.vi"("menu reference"=w135, "Command"=w137, "error in (no error)"=w136, "EpiWrapper in"=w140) -> ("error out"=w139:errorcluster, "EpiWrapper out"=w138:refnum<class "EpiWrapper.lvclass">)  [unwired: 6 in]
                  }
                  frame Enabled {
                    n92 = call-dynamic "MoveCurrentToSelected.vi"("error in (no error)"=w143, "EpiWrapper in"=w144) -> ("error out"=w142:errorcluster, "EpiWrapper out"=w141:refnum<class "EpiWrapper.lvclass">)  [unwired: 8 in]
                  }
                }
                n93 = flat-sequence {
                  tunnel: w131 -> [w145]
                  tunnel: [w146] -> w130
                  tunnel: w129 -> [w146]
                  tunnel: [w145] -> w125
                  frame #0 {
                    n94 = local write "Status"(FALSE ("Status")) -> ()
                  }
                }
              }
              frame "NEW" {
                n95 = call "NewWafer_Dial.vi"("error in (no error)"=w154) -> ("Cancelled?"=w159:bool, "StartLotTraveler"=w158:T30, "error out"=w153:errorcluster)  [unwired: 3 in]
                n96 = case shown="False" w159 {
                  tunnel: w158 -> [w160 _]
                  tunnel: w157 -> [w166 w168]
                  tunnel: w153 -> [w165 w167]
                  tunnel: [w164 w168] -> w156
                  tunnel: [w163 w167] -> w155
                  tunnel: w151 -> [w162 _]
                  tunnel: w152 -> [w161 _]
                  frame False {
                    n97 = call-dynamic "Prompting.vi"("menu reference"=w161, "Command"=w162, "error in (no error)"=w165, "StartLotTraveler"=w160, "EpiWrapper in"=w166) -> ("error out"=w163:errorcluster, "EpiWrapper out"=w164:refnum<class "EpiWrapper.lvclass">)  [unwired: 5 in]
                  }
                  frame True {
                  }
                }
              }
              frame "SAVE" {
                n98 = call-dynamic "Disable_Enable.vi"("menu reference"=w169, "Disabled"=T27."Enabled", "error in (no error)"=w178, "Command"=w170, "EpiWrapper in"=w179) -> ("error out"=w175:errorcluster, "EpiWrapper out"=w176:refnum<class "EpiWrapper.lvclass">)  [unwired: 5 in]
                n99 = call-dynamic "SaveLotData.vi"("error in (no error)"=w175, "EpiWrapper in"=w176) -> ("error out"=w173:errorcluster, "EpiWrapper out"=w174:refnum<class "EpiWrapper.lvclass">)  [unwired: 8 in]
                n100 = flat-sequence {
                  tunnel: [w181] -> w172
                  tunnel: w173 -> [w181]
                  tunnel: [w180] -> w171
                  tunnel: w174 -> [w180]
                  frame #0 {
                    n101 = One Button Dialog(message="Save Done") -> ()  [unwired: 1 in, 1 out]
                  }
                }
              }
              frame "SWAP_MODE" {
              }
              frame "UPDATE_ACQ" {
              }
              frame "EXIT" {
                n102 = disable-structure shown="Enabled" {
                  disable-tunnel: w190 -> [w195 w197]
                  disable-tunnel: w189 -> [w194 w196]
                  disable-tunnel: [w193 w197] -> w188
                  disable-tunnel: [w192 w196] -> w187
                  frame Enabled {
                    n103 = call-dynamic "Close.vi"("error in (no error)"=w194, "EpiWrapper in"=w195) -> ("error out"=w192:errorcluster, "EpiWrapper out"=w193:refnum<class "EpiWrapper.lvclass">)  [unwired: 8 in]
                  }
                  frame Disabled {
                  }
                }
              }
              frame "CANCEL" {
                n104 = call-dynamic "Prompting.vi"("menu reference"=w198, "Command"=w199, "error in (no error)"=w202, "EpiWrapper in"=w203) -> ("error out"=w201:errorcluster, "EpiWrapper out"=w200:refnum<class "EpiWrapper.lvclass">)  [unwired: 6 in]
              }
              frame "UPDATE_INT" {
                n105 = call-dynamic "UpdateIntegration.vi"("error in (no error)"=w206, "EpiWrapper in"=w207) -> ("error out"=w204:errorcluster, "EpiWrapper out"=w205:refnum<class "EpiWrapper.lvclass">)  [unwired: 1 in]
              }
              frame "RESET" {
                n106 = call-dynamic "Disable_Enable.vi"("menu reference"=w209, "Disabled"=T27."Disabled and Grayed Out", "error in (no error)"=w219, "Command"=Command_Enum."INIT", "EpiWrapper in"=w220) -> ("error out"=w216:errorcluster, "EpiWrapper out"=w217:refnum<class "EpiWrapper.lvclass">)  [unwired: 5 in]
                n107 = call-dynamic "Close.vi"("error in (no error)"=w216, "EpiWrapper in"=w217) -> ("error out"=w214:errorcluster, "EpiWrapper out"=w215:refnum<class "EpiWrapper.lvclass">)  [unwired: 8 in]
                n108 = call-dynamic "ProgInit.vi"("error in (no error)"=w214, "Intialize?"=FALSE, "EpiWrapper in"=w215) -> ("error out"=w212:errorcluster, "EpiWrapper out"=w213:refnum<class "EpiWrapper.lvclass">)  [unwired: 1 in]
                n109 = flat-sequence {
                  tunnel: [w223] -> w211
                  tunnel: w212 -> [w223]
                  tunnel: [w222] -> w210
                  tunnel: w213 -> [w222]
                  frame #0 {
                    n110 = One Button Dialog(message="Initialization Done") -> ()  [unwired: 1 in, 1 out]
                  }
                }
              }
              frame "OPENCONFIG" {
                n111 = call-dynamic "PromptConfig.vi"("error in (no error)"=w225, "EpiWrapper in"=w228) -> ("error out"=w227:errorcluster, "EpiWrapper out"=w226:refnum<class "EpiWrapper.lvclass">)
              }
              frame "RESETCONFIG" {
                n112 = call-dynamic "ResetConfiguration.vi"("error in (no error)"=w231, "EpiWrapper in"=w232) -> ("error out"=w230:errorcluster, "EpiWrapper out"=w229:refnum<class "EpiWrapper.lvclass">)
              }
              frame "SPECTRUMCAPTURE" {
                n113 = call-dynamic "Prompting.vi"("menu reference"=w233, "Command"=w234, "error in (no error)"=w237, "EpiWrapper in"=w238) -> ("error out"=w236:errorcluster, "EpiWrapper out"=w235:refnum<class "EpiWrapper.lvclass">)  [unwired: 6 in]
              }
              frame "INSITUMEASURE" {
                n114 = call-dynamic "Prompting.vi"("menu reference"=w240, "Command"=w239, "error in (no error)"=w241, "EpiWrapper in"=w244) -> ("error out"=w242:errorcluster, "EpiWrapper out"=w243:refnum<class "EpiWrapper.lvclass">)  [unwired: 6 in]
              }
              frame "MARK_MAP" {
                n115 = Variant To Data(error in=w252, type=cluster{"X":i32, "Y":i32} {"X"=0, "Y"=0} ("Mouse Position"), Variant=w253) -> (data=w247:cluster{"X":i32, "Y":i32}, error out=w248:errorcluster)
                n116 = call "Mark_Clicked_Selected.vi"("Coords"=w247, "error in (no error)"=w248, "EventType"=MapEventType."MouseClick", "EpiWrapper in"=w250) -> ("error out"=w245:errorcluster, "EpiWrapper out"=w246:refnum<class "EpiWrapper.lvclass">)  [unwired: 4 in]
              }
              frame "MARK_MAP_SELECT" {
                n117 = Variant To Data(error in=w262, type="" ("NewVal"), Variant=w261) -> (data=w257:string, error out=w258:errorcluster)
                n118 = call "Mark_Clicked_Selected.vi"("error in (no error)"=w258, "EventType"=MapEventType."DropDown", "Id"=w257, "EpiWrapper in"=w259) -> ("error out"=w254:errorcluster, "EpiWrapper out"=w255:refnum<class "EpiWrapper.lvclass">)  [unwired: 4 in]
              }
            }
          }
          frame Error {
            n119 = call <vilib>:"Clear Errors.vi"("error in (no error)"=w264) -> ("error out"=w263:errorcluster)  [unwired: 6 in]
          }
        }
        n120 = global read "Exit.vi" "Exit?"() -> (w74:bool)
        n121 = Or(x=w72, y=w74) -> (x .or. y?=w73:bool)
      }
      n122 = Release Queue(queue=w60, error in (no error)=w59) -> (error out=w58:errorcluster)  [unwired: 1 in, 2 out]
      n123 = Merge Errors(w56, w58) -> (w57:errorcluster)
      n124 = call <vilib>:"Clear Errors.vi"("error in (no error)"=w57) -> ()  [unwired: 6 in, 1 out]
    }
  }
  n125 = disable-structure shown="Disabled" {
    frame Disabled {
      (unwired) 0 ("X")
      (unwired) 0 ("Y")
      n126 = Variant To Data() -> (data=w362:T31, error out=w369:errorcluster)  [unwired: 3 in]
      n127 = call-dynamic "CheckClick.vi"("Enum"=enum16{"MouseClick", "DropDown"}."MouseClick", "error in (no error)"=w369, "Coords"=w362) -> ("error out"=w366:errorcluster, "OnPad?"=w363:bool, "Selected?"=w370:bool, "EpiWrapper out"=w365:refnum<class "EpiWrapper.lvclass">, "Id"=w364:string)  [unwired: 4 in]
      n128 = case shown="True" w363 {
        tunnel: w364 -> [_ w379]
        tunnel: w365 -> [w373 w380]
        tunnel: w366 -> [w372 w377]
        tunnel: [w372 w376] -> w367
        tunnel: [w373 w375] -> w368
        tunnel: w370 -> [_ w374]
        frame False {
        }
        frame True {
          n129 = Select(t=enum16{"Remove", "Mark", "Clear All"}."Remove" ("Enum"), s=w374, f=enum16{"Remove", "Mark", "Clear All"}."Mark" ("Enum")) -> (s? t:f=w378:enum16{"Remove", "Mark", "Clear All"})
          n130 = call "Mark_Clicked_Selected.vi"("error in (no error)"=w377, "Enum"=w378, "Id"=w379, "EpiWrapper in"=w380) -> ("error out"=w376:errorcluster, "EpiWrapper out"=w375:refnum<class "EpiWrapper.lvclass">)  [unwired: 2 in]
        }
      }
    }
    frame Enabled {
    }
  }
  n131 = disable-structure shown="Disabled" {
    disable-tunnel: w23 -> [w383 _]
    frame Disabled {
      n132 = Quit LabVIEW(quit? (T)=w383) -> ()
    }
    frame Enabled {
    }
  }
